vi "negate test.vi"() -> ()   [LabVIEW 2018]
uses:
  <vilib>/rvi/FXPMathLib/FxpConvert/subVIs/nifxpmath_Convert_SimConfig.ctl
  <vilib>/fxp/LVFixedPointQuantizationPolicyTypeDef.ctl
  <vilib>/fxp/LVFixedPointOverflowPolicyTypeDef.ctl
  <vilib>/rvi/FXPMathLib/FxpConvert/simVIs/DllFxpConvertTemp_sub.vi
  <vilib>/rvi/FXPMathLib/FxpConvert/XNode/nifxpmath_Convert.xnode
  <vilib>/rvi/FXPMathLib/FxpSub/XNode/nifxpmath_Sub.xnode
  <vilib>/rvi/FXPMathLib/sim/FxpSim.dll
panel:
  out "average 4":fxp<+/-,16,14> format="%016b"
  out "average 5":fxp<+/-,16,14>
  out "average 3":fxp<+/-,16,14> format="%016b"
  in  "average 2":fxp<+/-,16,14>
  out "average":fxp<+/-,16,14>
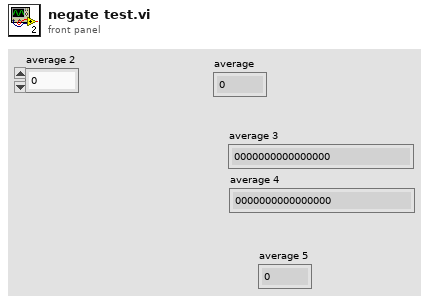
[diagram p1: front panel]
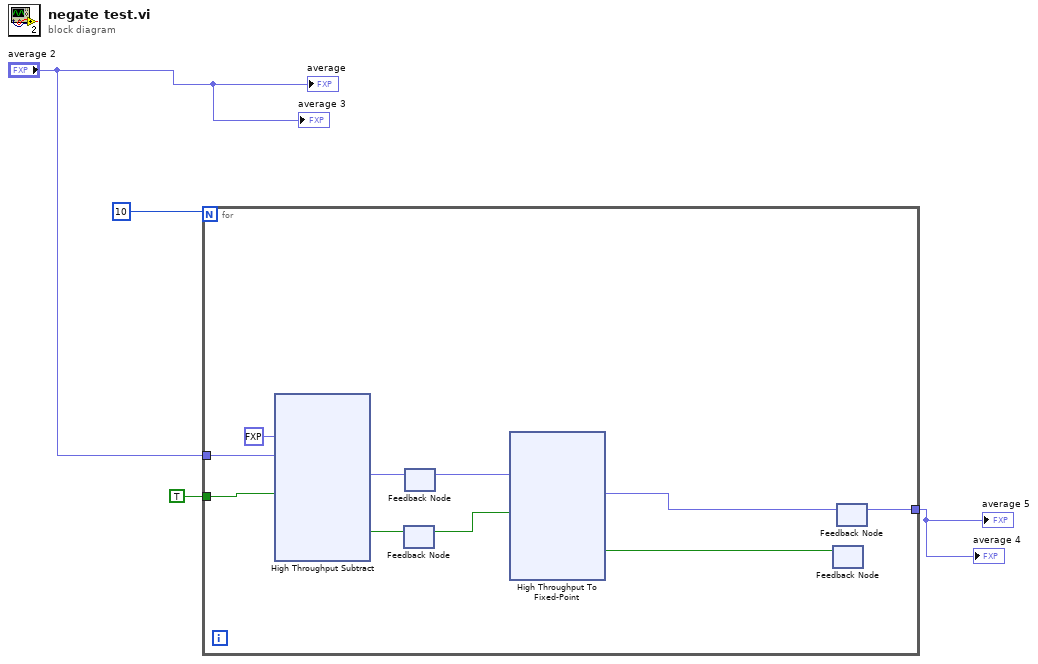
[diagram p0: block diagram]
diagram:
  n1 = for {
    N: 10 -> [_]
    tunnel: TRUE ("input valid") -> [w7]
    tunnel: "average 2" -> [w10]
    tunnel: [w12] -> w2
    n2 = xnode "High Throughput Subtract"("x"=fxp<+/-,16,14> 0.0, "y"=w10, "input valid"=w7) -> ("x-y"=w9:fxp<+/-,17,15>, "output valid"=w8:bool)  [unwired: 1 in, 1 out]
    n3 = feedback #1() -> (w14:bool)  [unwired: 1 in]
    n4 = feedback-in #1(w8) -> ()
    n5 = feedback #2() -> (w6:fxp<+/-,17,15>)  [unwired: 1 in]
    n6 = feedback-in #2(w9) -> ()
    n7 = xnode "High Throughput To Fixed-Point"("x"=w6, "input valid"=w14) -> ("y"=w5:fxp<+/-,16,14>, "output valid"=w13:bool)  [unwired: 1 in, 1 out]
    n8 = feedback #3() -> ()  [unwired: 2 in]
    n9 = feedback-in #3(w13) -> ()
    n10 = feedback #4() -> (w12:fxp<+/-,16,14>)  [unwired: 1 in]
    n11 = feedback-in #4(w5) -> ()
  }
  "average 5" <- w2
  "average 4" <- w2
  "average" <- "average 2"
  "average 3" <- "average 2"
